vi "Exp_ICCD_SetRepetitiveGateProperties.vi"(8 "error in (no error)":errorcluster, 9 "Repetitive Gate Width (ns)":dbl, 10 "Repetitive Gate Delay (ns)":dbl, 11 "LightField Automation in":refnum<class "LightField Automation.lvclass">) -> (0 "error out":errorcluster, 3 "LightField Automation out":refnum<class "LightField Automation.lvclass">)   [LabVIEW 2013, in "LightField Automation.lvclass"]
uses:
  LightField Automation.lvclass
  C:/Program Files/Princeton Instruments/LightField/AddInViews/PrincetonInstruments.LightFieldViewV3.dll
  Program Files/Princeton Instruments/LightField/AddInViews/PrincetonInstruments.LightFieldViewV3.dll
  C:/Program Files/Princeton Instruments/LightField/PrincetonInstruments.LightFieldAddInSupportServices.dll
  Program Files/Princeton Instruments/LightField/PrincetonInstruments.LightFieldAddInSupportServices.dll
  LightField Automation.lvclass/LightField Automation.ctl
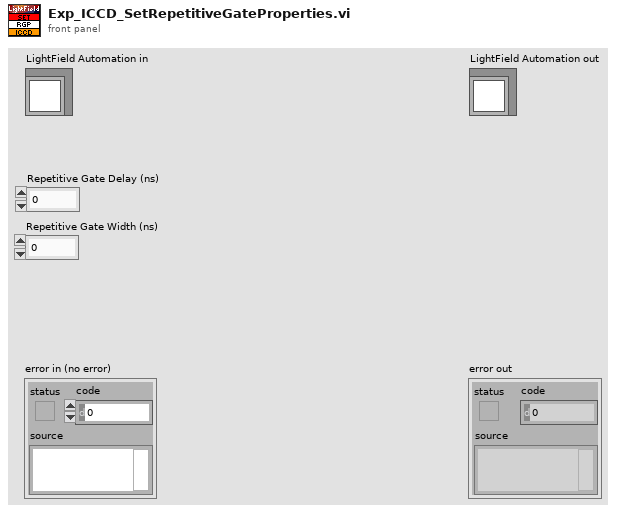
[diagram p1: front panel]
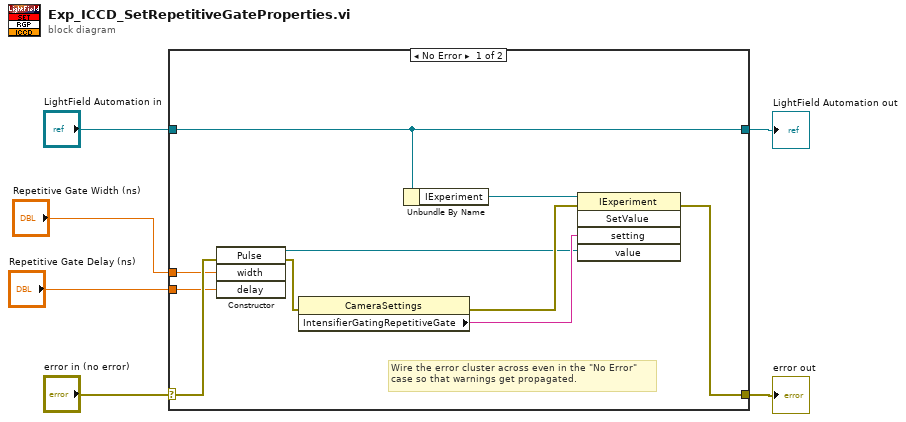
[diagram p0: block diagram]
diagram:
  n1 = case shown="No Error" "error in (no error)" {
    selector: "error in (no error)" -> [w10 w18]
    tunnel: [w15 w18] -> w5
    tunnel: [w16 w17] -> w3
    tunnel: "LightField Automation in" -> [w16 w17]
    tunnel: "Repetitive Gate Width (ns)" -> [w8 _]
    tunnel: "Repetitive Gate Delay (ns)" -> [w7 _]
    frame No Error {
      # "Wire the error cluster across even in the \"No Error\"\ncase so that warnings get propagated."
      n2 = constructor class="Pulse"(error in=w10, "width"=w8, "delay"=w7) -> (reference out=w11:refnum<k24>, error out=w9:errorcluster)  [unwired: 2 in, 3 out]
      n3 = property class="CameraSettings"(error in=w9) -> (error out=w12:errorcluster, "IntensifierGatingRepetitiveGate"=w13:string)  [unwired: 1 in, 1 out]
      n4 = Unbundle By Name(w16) -> ("IExperiment"=w14:refnum<k24>)
      n5 = invoke class="IExperiment" method="SetValue"(reference=w14, error in=w12, "setting"=w13, "value"=w11) -> (error out=w15:errorcluster)  [unwired: 1 in, 4 out]
    }
    frame Error {
    }
  }
  "error out" <- w5
  "LightField Automation out" <- w3
